vi "getData.vi"() -> (3 "output array":cluster{"Degree":dbl, "Magnitude":dbl}[](array[cluster]))   [LabVIEW 2014]
uses:
  Robot Global Data.vi
  <vilib>/Rock Robotics/Network Tables/SD Read Number.vi
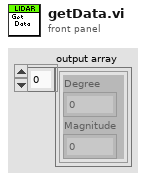
[diagram p1: front panel]
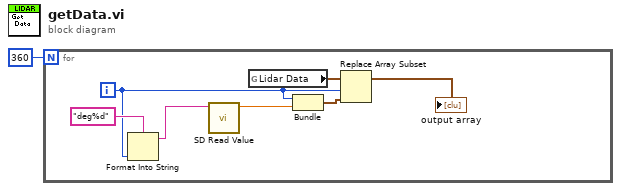
[diagram p0: block diagram]
diagram:
  n1 = for {
    N: 360 -> [_]
    i -> [w6]
    n2 = Format Into String(format string="deg%d", w6) -> (resulting string=w7:string)  [unwired: 2 in, 1 out]
    n3 = call-poly <vilib>:"SD Read Value.vi"("Name"=w7) -> ("Numeric"=w3:dbl)  [unwired: 8 in, 2 out]
    n4 = global read "Robot Global Data.vi" "Lidar Data"() -> (w5:cluster{"Degree":dbl, "Magnitude":dbl}[])
    n5 = Bundle(w6, "Numeric"=w3) -> (w4:cluster{i32, "Numeric":dbl})  [unwired: 1 in]
    n6 = Replace Array Subset(array=w5, new element=w4, index=w6) -> (→"output array":cluster{"Degree":dbl, "Magnitude":dbl}[])
  }
